vi "AutoCreateFolder.vi"(8 "error in (no error)":errorcluster, 10 "Names":string[](array[string]), 11 "Base path":path) -> (0 "error out":errorcluster, 3 "Created path":path)   [LabVIEW 2020, in "Other.lvlib"]
uses:
  Other.lvlib
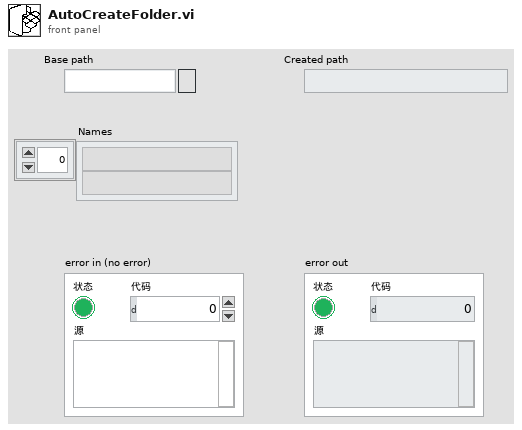
[diagram p1: front panel]
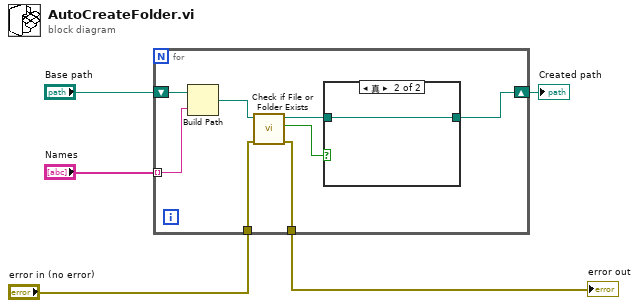
[diagram p0: block diagram]
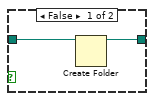
[diagram p2: hidden frame]
diagram:
  n1 = for {
    tunnel: "Names" -> [w12] mode=indexing
    shift-right: [w8] -> w1
    shift-left: "Base path" -> [w13]
    tunnel: "error in (no error)" -> [w7]
    tunnel: [w6] -> w2
    n2 = Build Path(base path=w13, name or relative path=w12) -> (appended path=w11:path)
    n3 = call <vilib>:"Check if File or Folder Exists.vi"("error in (no error)"=w7, "path"=w11) -> ("error out"=w6:errorcluster, "file or folder exists?"=w10:bool, "dup path"=w9:path)  [unwired: 7 in]
    n4 = case shown="真" w10 {
      tunnel: w9 -> [w15 w16]
      tunnel: [w14 w16] -> w8
      frame False {
        n5 = Create Folder(path (use dialog)=w15) -> (created path=w14:path)  [unwired: 2 in, 2 out]
      }
      frame True {
      }
    }
  }
  "error out" <- w2
  "Created path" <- w1
